vi "GLOBAL_BENCH.vi"() -> ()   [LabVIEW 2014]
panel:
  out "BENCH_PARAMS":T1
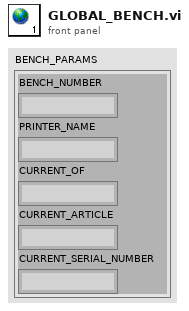
[diagram p1: front panel]
types:
  T1 = cluster{"BENCH_NUMBER":string, "PRINTER_NAME":string, "CURRENT_OF":string, "CURRENT_ARTICLE":string, "CURRENT_SERIAL_NUMBER":string}
diagram:
